vi "Calculate Executed Test Count.vi"(8 "Test Selector Array":bool[](array[boolean]), 9 "Multiplier of Runs":i32, 10 "All Test Count":i32, 11 "Run All Tests":bool) -> (3 "Executed Test Count":i32)   [LabVIEW 2018, in "Common Support.lvlib"]
uses:
  Common Support.lvlib
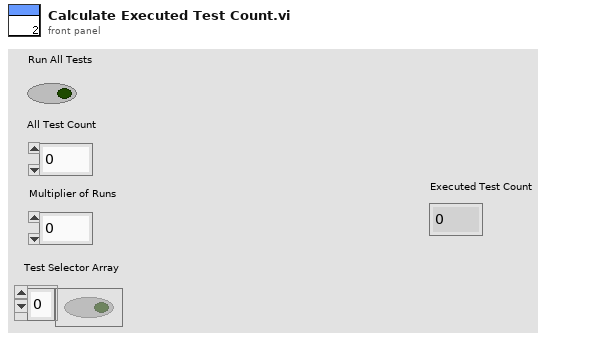
[diagram p1: front panel]
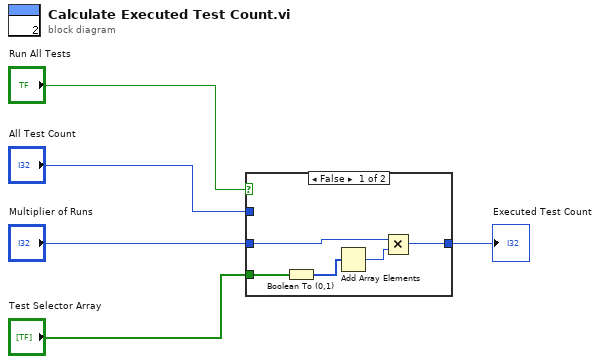
[diagram p0: block diagram]
diagram:
  n1 = case shown="False" "Run All Tests" {
    tunnel: [w7 w11] -> w3
    tunnel: "Test Selector Array" -> [w10 _]
    tunnel: "Multiplier of Runs" -> [w6 _]
    tunnel: "All Test Count" -> [_ w11]
    frame False {
      n2 = Boolean To (0,1)(Boolean=w10) -> (0, 1=w9:i16[])
      n3 = Add Array Elements(numeric array=w9) -> (sum=w8:i16)
      n4 = Multiply(x=w6, y=w8) -> (x*y=w7:i32)
    }
    frame True {
    }
  }
  "Executed Test Count" <- w3
